vi "Read Compensated Pressure from BMP-180.vi"(1 "CalCoeffs":dbl[](array[numeric])) -> (0 "Pressure":dbl)   [LabVIEW 2014]
panel:
  in  "Raw Temp":u16
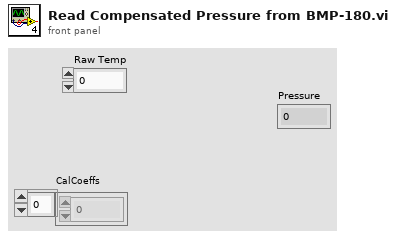
[diagram p1: front panel]
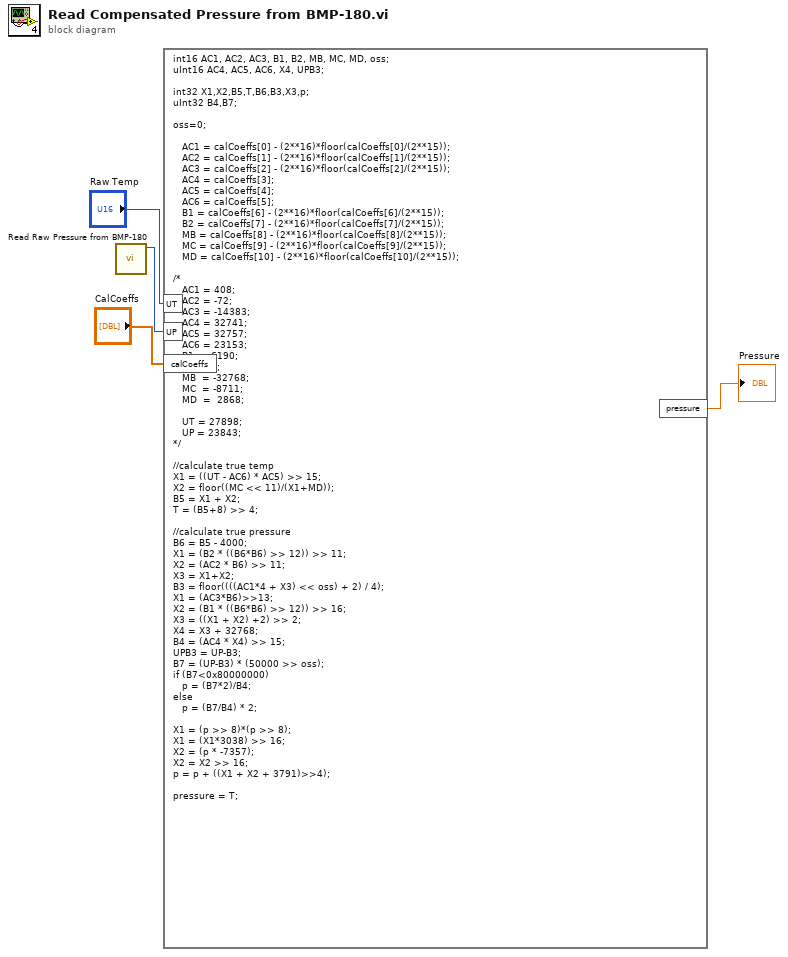
[diagram p0: block diagram]
diagram:
  n1 = call "Read Raw Pressure from BMP-180.vi"() -> ("Numeric"=w1:u16)  [unwired: 11 in]
  n2 = formula code="int16 AC1, AC2, AC3, B1, B2, MB, MC, MD, oss;\nuInt16 AC4, AC5, AC6, X4, UPB3;\n\nint32 X1,X2,B5,T,B6,B3,X3,p;\nuInt32 B4,B7;\n\noss=0;\n\n   AC1 = calCoeffs[0] - (2**16)*floor(calCoeffs[0]/(2**15));\n   AC2 = calCoeffs[1] - (2**16)*floor(calCoeffs[1]/(2**15));\n   AC3 = calCoeffs[2] - (2**16)*floor(calCoeffs[2]/(2**15));\n   AC4 = calCoeffs[3];\n   AC5 = calCoeffs[4];\n   AC6 = calCoeffs[5];\n   B1 = calCoeffs[6] - (2**16)*floor(calCoeffs[6]/(2**15));\n   B2 = calCoeffs[7] - (2**16)*floor(calCoeffs[7]/(2**15));\n   MB = calCoeffs[8] - (2**16)*floor(calCoeffs[8]/(2**15));\n   MC = calCoeffs[9] - (2**16)*floor(calCoeffs[9]/(2**15));\n   MD = calCoeffs[10] - (2**16)*floor(calCoeffs[10]/(2**15));\n\n/*\n   AC1 = 408;\n   AC2 = -72;\n   AC3 = -14383;\n   AC4 = 32741;\n   AC5 = 32757;\n   AC6 = 23153;\n   B1  = 6190;\n   B2  = 4;\n   MB  = -32768;\n   MC  = -8711;\n   MD  =  2868;\n\n   UT = 27898;\n   UP = 23843;  \n*/\n\n//calculate true temp\nX1 = ((UT - AC6) * AC5) >> 15;\nX2 = floor((MC << 11)/(X1+MD));\nB5 = X1 + X2;\nT = (B5+8) >> 4;\n\n//calculate true pressure\nB6 = B5 - 4000;\nX1 = (B2 * ((B6*B6) >> 12)) >> 11;\nX2 = (AC2 * B6) >> 11;\nX3 = X1+X2;\nB3 = floor((((AC1*4 + X3) << oss) + 2) / 4);\nX1 = (AC3*B6)>>13;\nX2 = (B1 * ((B6*B6) >> 12)) >> 16;\nX3 = ((X1 + X2) +2) >> 2;\nX4 = X3 + 32768;\nB4 = (AC4 * X4) >> 15;\nUPB3 = UP-B3;\nB7 = (UP-B3) * (50000 >> oss);\nif (B7<0x80000000)\n   p = (B7*2)/B4;\nelse\n   p = (B7/B4) * 2;\n\nX1 = (p >> 8)*(p >> 8);\nX1 = (X1*3038) >> 16;\nX2 = (p * -7357);\nX2 = X2 >> 16;\np = p + ((X1 + X2 + 3791)>>4);\n\npressure = T;"("UT"="Raw Temp", "UP"=w1, "calCoeffs"="CalCoeffs") -> ("pressure"=→"Pressure":dbl)
